vi "ODMR (external triggers).vi"() -> ()   [LabVIEW 2025]
uses:
  <vilib>/DAQmx/write.llb/DAQmx Write (Analog DBL 1Chan 1Samp).vi
  <vilib>/Analysis/1siggen.llb/Ramp Pattern by Samples.vi
  <vilib>/DAQmx/write.llb/DAQmx Write (Digital Bool 1Line 1Point).vi
  <vilib>/DAQmx/read.llb/DAQmx Read (Digital Bool 1Line 1Point).vi
  <vilib>/DAQmx/read.llb/DAQmx Read (Counter DBL 1Chan 1Samp).vi
  <vilib>/DAQmx/write.llb/DAQmx Write (Analog 1D DBL NChan 1Samp).vi
  <vilib>/DAQmx/create/channels.llb/DAQmx Create Channel (AO-Voltage-Basic).vi
  <vilib>/DAQmx/miscellaneous.llb/DAQmx Fill In Error Info.vi
  <vilib>/DAQmx/create/channels.llb/DAQmx Create Channel (DO-Digital Output).vi
  <vilib>/DAQmx/create/channels.llb/DAQmx Create Channel (DI-Digital Input).vi
  <vilib>/DAQmx/create/channels.llb/DAQmx Create Channel (CI-Count Edges).vi
  <vilib>/Analysis/NI_AALBase.lvlib
panel:
  out "data":bool
  out "XY Graph":cluster{"Y":dbl[], "Y":dbl[]}[](graph)
  in  "Dwell time (ms)":u32=30
  out "interations":i32
  in  "Vx":dbl
  in  "Vy":dbl
  in  "End frequency (Ghz)":dbl
  in  "start frequency (Ghz)":dbl
  in  "Step size (Mhz)":dbl
  in  "VISA resource name":refnum<visa-resource-name>
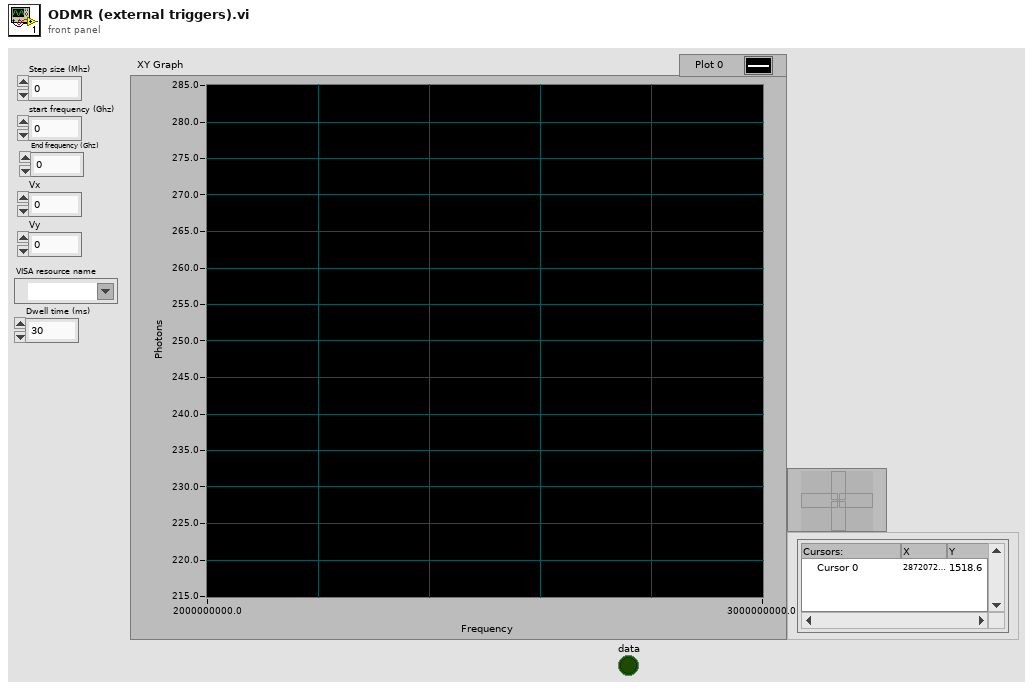
[diagram p1: front panel]
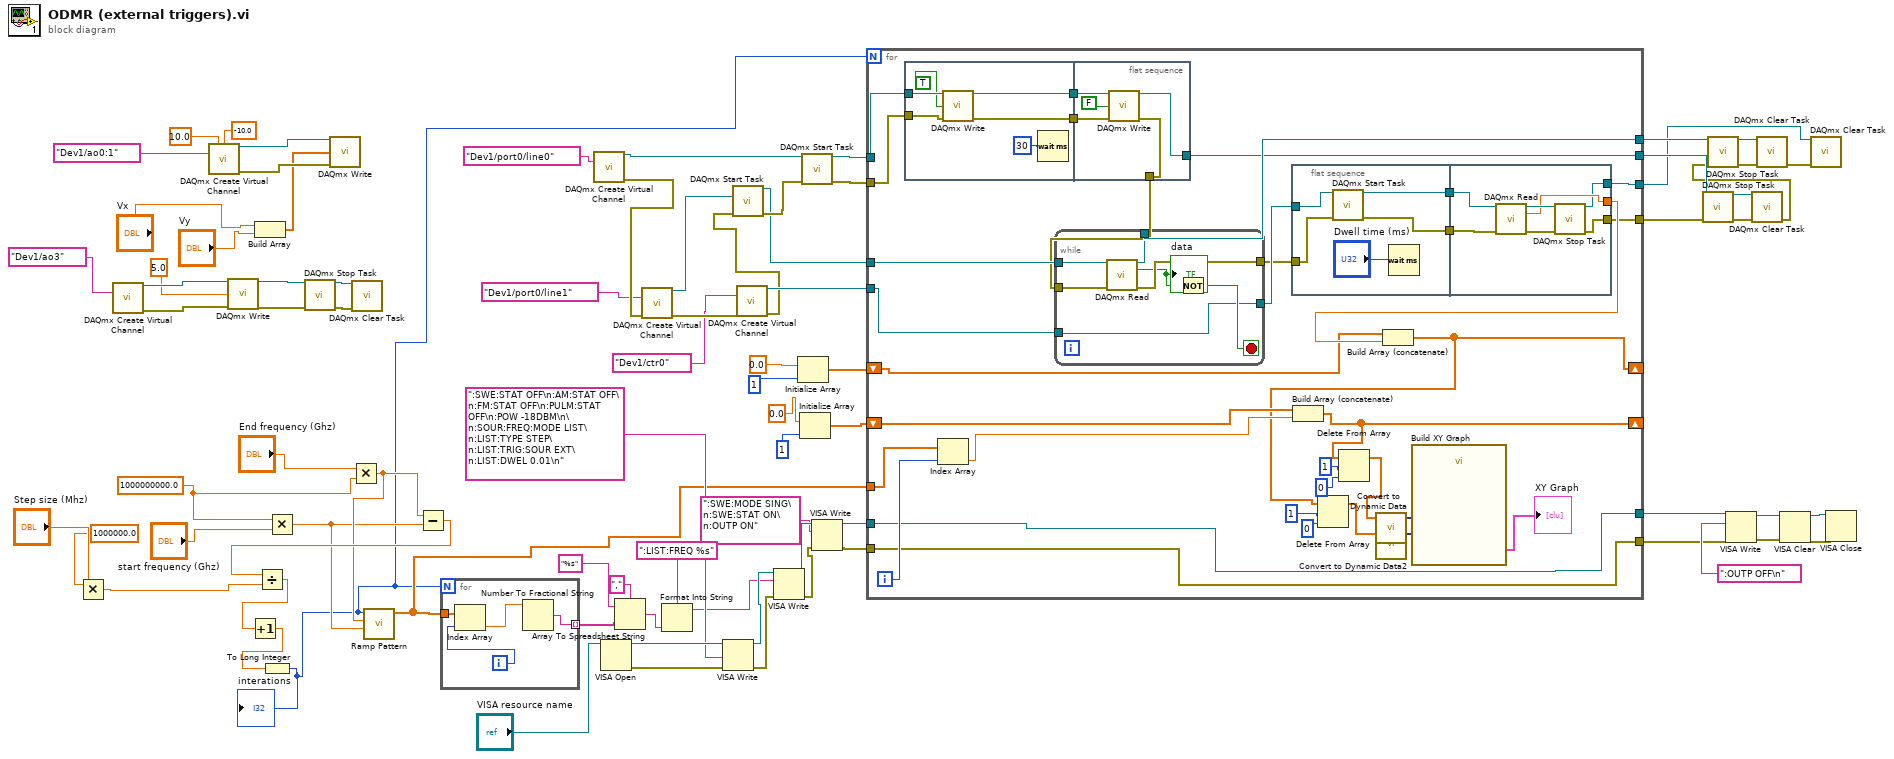
[diagram p0: block diagram]
diagram:
  w73 = 1000000000.0 ("x")
  n1 = Multiply(x=1000000.0, y="Step size (Mhz)") -> (x*y=w70:dbl)
  n2 = call-poly <vilib>:"DAQmx Create Virtual Channel.vi"("physical channels"=tag "Dev1/ao3") -> ("task out"=w60:refnum<k21>, "error out"=w61:errorcluster)  [unwired: 13 in]
  n3 = call-poly <vilib>:"DAQmx Create Virtual Channel.vi"("maximum value"=10.0, "minimum value"=-10.0, "physical channels"=tag "Dev1/ao0:1") -> ("task out"=w82:refnum<k21>, "error out"=w78:errorcluster)  [unwired: 11 in]
  n4 = call-poly <vilib>:"DAQmx Write.vi"("task/channels in"=w60, "data"=5.0, "error in"=w61) -> ("task out"=w56:refnum<k21>, "error out"=w58:errorcluster)  [unwired: 10 in, 1 out]
  n5 = Build Array("Vx", "Vy") -> (w69:dbl[])
  n6 = Multiply(x=w73, y="start frequency (Ghz)") -> (x*y=w52:dbl)
  n7 = call <vilib>:"DAQmx Stop Task.vi"("task/channels in"=w56, "error in"=w58) -> ("task out"=w55:refnum<k21>, "error out"=w57:errorcluster)  [unwired: 12 in]
  n8 = call-poly <vilib>:"DAQmx Write.vi"("task/channels in"=w82, "data"=w69, "error in"=w78) -> ()  [unwired: 10 in, 3 out]
  n9 = Multiply(x="End frequency (Ghz)", y=w73) -> (x*y=w53:dbl)
  n10 = call <vilib>:"DAQmx Clear Task.vi"("task in"=w55, "error in"=w57) -> ()  [unwired: 13 in, 1 out]
  n11 = Subtract(x=w53, y=w52) -> (x-y=w71:dbl)
  n12 = Divide(x=w71, y=w70) -> (x/y=w65:dbl)
  n13 = Increment(x=w65) -> (x+1=w54:dbl)
  n14 = To Long Integer(number=w54) -> (32bit integer=w11:i32)
  "interations" <- w11
  n15 = call-poly <vilib>:"Ramp Pattern.vi"("start"=w52, "end"=w53, "samples"=w11) -> ("Ramp Pattern"=w35:dbl[])  [unwired: 7 in, 1 out]
  n16 = for {
    N: w11 -> [_]
    tunnel: w35 -> [w86]
    tunnel: [w83] -> w10 mode=indexing
    i -> [w85]
    n17 = Index Array(array=w86, index=w85) -> (element=w84:dbl)
    n18 = Number To Fractional String(number=w84) -> (F-format string=w83:string)  [unwired: 3 in]
  }
  n19 = call-poly <vilib>:"DAQmx Create Virtual Channel.vi"("lines"=tag "Dev1/port0/line0") -> ("task out"=w50:refnum<k21>, "error out"=w45:errorcluster)  [unwired: 13 in]
  n20 = VISA Open(VISA resource name="VISA resource name") -> (VISA resource name=w79:refnum<visa-resource-name>, error out=w77:errorcluster)  [unwired: 4 in]
  n21 = Array To Spreadsheet String(delimiter (Tab)=",", array=w10, 3:"%s" ("format string")) -> (spreadsheet string=w8:string)
  n22 = call-poly <vilib>:"DAQmx Create Virtual Channel.vi"("lines"=tag "Dev1/port0/line1", "error in"=w45) -> ("task out"=w46:refnum<k21>, "error out"=w14:errorcluster)  [unwired: 12 in]
  n23 = Format Into String(format string=":LIST:FREQ %s", w8) -> (resulting string=w2:string)  [unwired: 2 in, 1 out]
  n24 = VISA Write(VISA resource name=w79, write buffer=":SWE:STAT OFF\n:AM:STAT OFF\n:FM:STAT OFF\n:PULM:STAT OFF\n:POW -18DBM\n\n:SOUR:FREQ:MODE LIST\n:LIST:TYPE STEP\n:LIST:TRIG:SOUR EXT\n:LIST:DWEL 0.01\n", error in (no error)=w77) -> (VISA resource name out=w6:refnum<visa-resource-name>, error out=w5:errorcluster)  [unwired: 1 out]
  n25 = call-poly <vilib>:"DAQmx Create Virtual Channel.vi"("counter"=tag "Dev1/ctr0", "error in"=w14) -> ("task out"=w42:refnum<k21>, "error out"=w15:errorcluster)  [unwired: 12 in]
  n26 = call <vilib>:"DAQmx Start Task.vi"("task/channels in"=w46, "error in"=w15) -> ("task out"=w43:refnum<k21>, "error out"=w44:errorcluster)  [unwired: 12 in]
  n27 = VISA Write(VISA resource name=w6, write buffer=w2, error in (no error)=w5) -> (VISA resource name out=w4:refnum<visa-resource-name>, error out=w3:errorcluster)  [unwired: 1 out]
  n28 = Initialize Array(0.0 ("element"), 1 ("dimension size")) -> (w39:dbl[])
  n29 = Initialize Array(0.0 ("element"), 1 ("dimension size")) -> (w36:dbl[])
  n30 = call <vilib>:"DAQmx Start Task.vi"("task/channels in"=w50, "error in"=w44) -> ("task out"=w49:refnum<k21>, "error out"=w48:errorcluster)  [unwired: 12 in]
  n31 = VISA Write(VISA resource name=w4, write buffer=":SWE:MODE SING\n:SWE:STAT ON\n:OUTP ON", error in (no error)=w3) -> (VISA resource name out=w18:refnum<visa-resource-name>, error out=w16:errorcluster)  [unwired: 1 out]
  n32 = for {
    N: w11 -> [_]
    tunnel: w49 -> [w120]
    tunnel: w48 -> [w119]
    tunnel: w43 -> [w118]
    tunnel: w42 -> [w117]
    shift-right: [w98] -> _
    shift-left: w39 -> [w111]
    shift-right: [w97] -> _
    shift-left: w36 -> [w110]
    tunnel: w35 -> [w108]
    tunnel: [w88] -> w32
    tunnel: [w95] -> w29
    tunnel: [w94] -> w27
    tunnel: [w93] -> w26
    tunnel: [w92] -> w19
    tunnel: w18 -> [w92]
    tunnel: [w91] -> w17
    tunnel: w16 -> [w91]
    i -> [w109]
    n33 = flat-sequence {
      tunnel: w120 -> [w126]
      tunnel: w119 -> [w125]
      tunnel: [w124] -> w90
      tunnel: [w123] -> w89
      tunnel: w90 -> [w131]
      tunnel: w89 -> [w130]
      tunnel: [w129] -> w88
      tunnel: [w128] -> w87
      frame #0 {
        n34 = call-poly <vilib>:"DAQmx Write.vi"("task/channels in"=w126, "data"=TRUE, "error in"=w125) -> ("task out"=w124:refnum<k21>, "error out"=w123:errorcluster)  [unwired: 10 in, 1 out]
        n35 = Wait (ms)(milliseconds to wait=u32 30) -> ()  [unwired: 1 out]
      }
      frame #1 {
        n36 = call-poly <vilib>:"DAQmx Write.vi"("task/channels in"=w131, "data"=FALSE, "error in"=w130) -> ("task out"=w129:refnum<k21>, "error out"=w128:errorcluster)  [unwired: 10 in, 1 out]
      }
    }
    n37 = Index Array(array=w108, index=w109) -> (element=w107:dbl)
    n38 = while {
      tunnel: w118 -> [w150]
      tunnel: w87 -> [w149]
      tunnel: w117 -> [w147]
      tunnel: [w147] -> w116
      tunnel: [w146] -> w115
      tunnel: [w145] -> w94
      stop <- w148 stop-if-true
      n39 = call-poly <vilib>:"DAQmx Read.vi"("task/channels in"=w150, "error in"=w149) -> ("task out"=w145:refnum<k21>, "data"=w144:bool, "error out"=w146:errorcluster)  [unwired: 11 in]
      "data" <- w144
      n40 = Not(x=w144) -> (.not. x?=w148:bool)
    }
    n41 = flat-sequence {
      tunnel: w116 -> [w135]
      tunnel: w115 -> [w136]
      tunnel: [w133] -> w114
      tunnel: [w132] -> w113
      tunnel: w114 -> [w141]
      tunnel: w113 -> [w140]
      tunnel: [w139] -> w112
      tunnel: [w138] -> w95
      tunnel: [w137] -> w93
      frame #0 {
        n42 = call <vilib>:"DAQmx Start Task.vi"("task/channels in"=w135, "error in"=w136) -> ("task out"=w132:refnum<k21>, "error out"=w133:errorcluster)  [unwired: 12 in]
        n43 = Wait (ms)(milliseconds to wait="Dwell time (ms)") -> ()  [unwired: 1 out]
      }
      frame #1 {
        n44 = call-poly <vilib>:"DAQmx Read.vi"("task/channels in"=w140, "error in"=w141) -> ("task out"=w142:refnum<k21>, "data"=w139:dbl, "error out"=w143:errorcluster)  [unwired: 11 in]
        n45 = call <vilib>:"DAQmx Stop Task.vi"("task/channels in"=w142, "error in"=w143) -> ("task out"=w137:refnum<k21>, "error out"=w138:errorcluster)  [unwired: 12 in]
      }
    }
    n46 = Build Array (concatenate)(w110, w107) -> (w97:dbl[])
    n47 = Delete From Array(array=w97, length=1, index=0) -> (array with subset deleted=w99:dbl[])  [unwired: 1 out]
    n48 = call "Convert to Dynamic Data"("Array"=w99) -> ("Dynamic Data Type"=w106:dynamicdata)  [unwired: 3 in]
    n49 = Build Array (concatenate)(w111, w112) -> (w98:dbl[])
    n50 = Delete From Array(array=w98, length=1, index=0) -> (array with subset deleted=w100:dbl[])  [unwired: 1 out]
    n51 = call "Convert to Dynamic Data2"("Array"=w100) -> ("Dynamic Data Type"=w105:dynamicdata)  [unwired: 3 in]
    n52 = call "Build XY Graph"("Y Input"=w105, "X Input"=w106) -> ("XY Graph"=→"XY Graph":cluster{"X":dbl[], "Y":dbl[]}[])  [unwired: 8 in, 1 out]
  }
  n53 = call <vilib>:"DAQmx Stop Task.vi"("task/channels in"=w32, "error in"=w29) -> ("task out"=w34:refnum<k21>, "error out"=w33:errorcluster)  [unwired: 12 in]
  n54 = VISA Write(VISA resource name=w19, write buffer=":OUTP OFF\n", error in (no error)=w17) -> (VISA resource name out=w21:refnum<visa-resource-name>, error out=w22:errorcluster)  [unwired: 1 out]
  n55 = call <vilib>:"DAQmx Clear Task.vi"("task in"=w34, "error in"=w33) -> ("error out"=w28:errorcluster)  [unwired: 13 in]
  n56 = call <vilib>:"DAQmx Stop Task.vi"("task/channels in"=w27, "error in"=w28) -> ("task out"=w31:refnum<k21>, "error out"=w30:errorcluster)  [unwired: 12 in]
  n57 = call <vilib>:"DAQmx Clear Task.vi"("task in"=w31, "error in"=w30) -> ("error out"=w25:errorcluster)  [unwired: 13 in]
  n58 = VISA Clear(VISA resource name=w21, error in (no error)=w22) -> (VISA resource name out=w24:refnum<visa-resource-name>, error out=w23:errorcluster)
  n59 = call <vilib>:"DAQmx Clear Task.vi"("task in"=w26, "error in"=w25) -> ()  [unwired: 13 in, 1 out]
  n60 = VISA Close(VISA resource name=w24, error in (no error)=w23) -> ()  [unwired: 1 out]
